vi "Channel Measurement Fetch Memory Formatted.vi"(8 "error in (no error)":errorcluster {"code" format="%.0x"}, 9 "RetValBufferSize":i32=2048, 10 "RepCapIdentifier":string, 11 "instrument handle":refnum<k15>) -> (0 "error out":errorcluster {"code" format="%.0x"}, 1 "RetValActualSize":i32, 2 "RetVal":dbl[](array[numeric]) format="%.2p", 3 "instrument handle out":refnum<k15>)   [LabVIEW 2014, in "Agilent NA.lvlib"]
doc: "Returns measurement data in the current format as set by the Measurement.Format property. Smith and Polar formats are not supported."
uses:
  Agilent NA.lvlib
  AgNA.dll
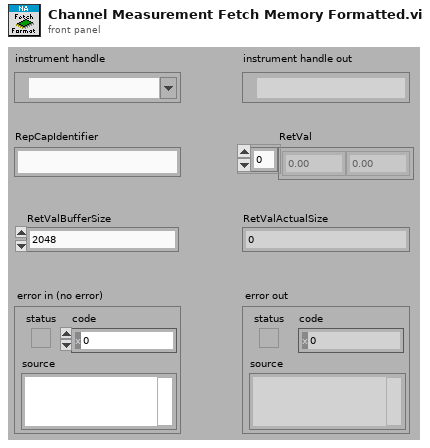
[diagram p1: front panel]
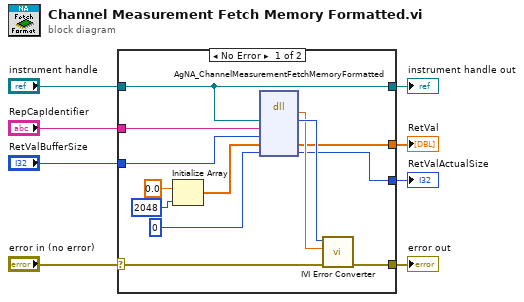
[diagram p0: block diagram]
diagram:
  n1 = case shown="No Error" "error in (no error)" {
    selector: "error in (no error)" -> [w19 w23]
    tunnel: [w18 w23] -> w8
    tunnel: "RepCapIdentifier" -> [w17 _]
    tunnel: "RetValBufferSize" -> [w16 _]
    tunnel: [w12 _] -> w4
    tunnel: [w10 _] -> w3
    tunnel: [w9 w22] -> w2
    tunnel: "instrument handle" -> [w9 w22]
    frame No Error {
      n2 = Initialize Array(0.0 ("element"), 2048 ("dimension size")) -> (w15:dbl[])
      n3 = dll-call lib="AgNA**.dll" fn="AgNA_ChannelMeasurementFetchMemoryFormatted"("Vi"=w9, "RepCapIdentifier"=w17, "RetValBufferSize"=w16, "RetVal"=w15, "RetValActualSize"=0) -> ("return type"=w20:sgl, "Vi"=w21:u32, "RetVal"=w12:sgl[], "RetValActualSize"=w10:i32)  [unwired: 5 in, 2 out]
      n4 = call "IVI Error Converter.vi"("error in (no error)"=w19, "IVI error code (0)"=w20, "instrument handle"=w21) -> ("error out"=w18:errorcluster)  [unwired: 7 in, 1 out]
    }
    frame Error {
    }
  }
  "error out" <- w8
  "instrument handle out" <- w2
  "RetVal" <- w4
  "RetValActualSize" <- w3
